vi "State_Machine.vi"(8 "error in (no error)":errorcluster caption="entrée d'erreur (pas d'erreur)", 11 "Get_Voltage en entrée":refnum<class "Get_SN_DB_AIS.lvclass">) -> (0 "error out":errorcluster caption="sortie d'erreur", 2 "Json_String":string, 3 "Get_Voltage en sortie":refnum<class "Get_SN_DB_AIS.lvclass">)   [LabVIEW 2020, in "Library Test.lvlib" / "Get_SN_DB_AIS.lvclass"]
uses:
  Get_SN_DB_AIS.lvclass
  C:/Users/ngarcin/OneDrive - Altyor/Standard TB/Suite TB45/Class/Test/Test (Default)/Test (Default).lvclass
  Database/Database Altyor/Database Altyor.lvclass
  C:/Users/ngarcin/OneDrive - Altyor/Standard TB/Suite TB45/Class/Database/Database drivers/Database Drivers.lvclass
  Commun VI/TypeDef/Variable Printable.ctl
  JSON API/JSON Value/Set from JSON string.vi
  Instrument/Instrument (Default)/Class Instrument (Default).lvclass
  JSON API/JSON Value/JSON Value.lvclass
  JSON API/Variant JSON/Variant JSON.lvlib
  JSON API/Get Polymorphic/JSON GetSet.lvlib
  Commun VI/Library Commun.lvlib
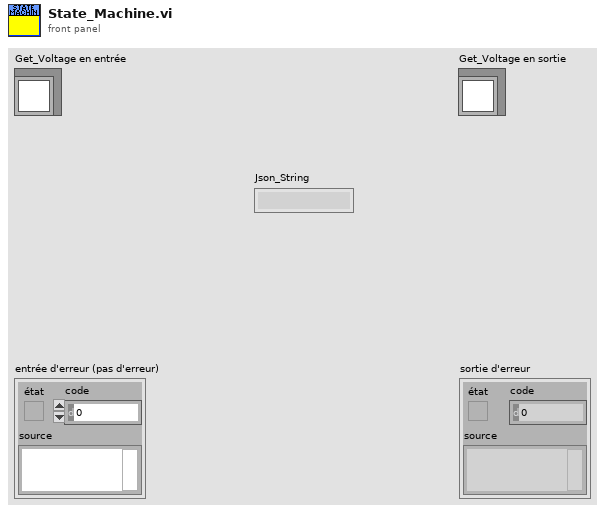
[diagram p1: front panel]
types:
  T1 = typedef "Variable Printable.ctl" = string
  T2 = enum16{"Get Variable", "Get All Variables", "Set Variable", "Delete Variable", "Delete All Variable"}
  T3 = cluster{"Connection Name ODBC":string, "DatabaseName":string, "Condition":string, "Type Data ":enum16{"Data Product", "Data Test"}, "Database Altyor":refnum<class "Database Altyor.lvclass">}
  T4 = cluster{"idTest":u32, "CreationDate":string, "EndOfProduction":string, "OrderNumber":string, "Batch":string, "ProductName":string, "PartNumber":string, "SerialNumber":string, "Operator":string, "Result":string, "AdditionalInformation":string}[]
  T5 = cluster{"idTest":u32, "CreationDate":string, "EndOfProduction":string, "OrderNumber":string, "Batch":string, "ProductName":string, "PartNumber":string, "SerialNumber":string, "Operator":string, "Result":string, "AdditionalInformation":string}
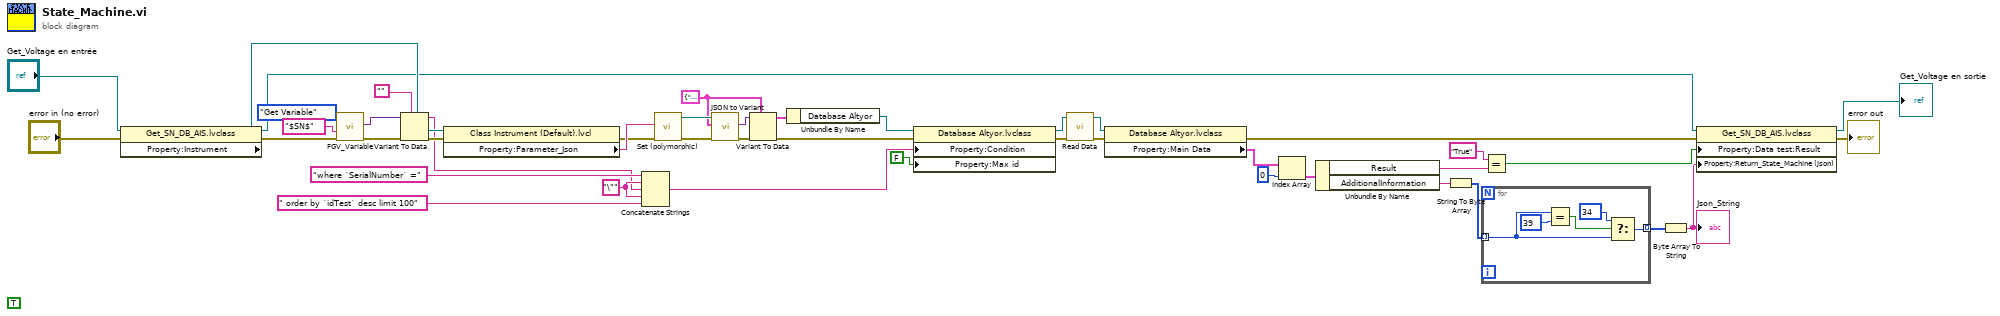
[diagram p0: block diagram]
diagram:
  w18 = "\"" ("chaîne")
  (unwired) TRUE ("Max id")
  w40 = T3 {"Connection Name ODBC"="", "DatabaseName"="", "Condition"="", "Type Data "=enum."Data Product", "Database Altyor"=refnum} ("Parameter")
  n1 = property class="Get_SN_DB_AIS.lvclass"(reference="Get_Voltage en entrée", error in="error in (no error)") -> (reference out=w9:refnum<class "Get_SN_DB_AIS.lvclass">, error out=w25:errorcluster, "Property:Instrument"=w23:refnum<class "Class Instrument (Default).lvclass">)
  n2 = call "FGV_Variable.vi"("error in (no error)"=w25, "Variable"=T1 "$SN$", "Function"=T2."Get Variable") -> ("error out"=w24:errorcluster, "Data Out"=w22:variant)  [unwired: 6 in, 1 out]
  n3 = Variant To Data(error in=w24, type="", Variant=w22) -> (data=w17:string, error out=w21:errorcluster)
  n4 = property class="Class Instrument (Default).lvcl"(reference=w23, error in=w21) -> (error out=w38:errorcluster, "Property:Parameter_Json"=w39:string)  [unwired: 1 out]
  n5 = Concatenate Strings("where `SerialNumber` =" ("chaîne"), w18, w17, w18, " order by `idTest` desc limit 100" ("chaîne")) -> (w16:string)
  n6 = call-poly "Set (polymorphic).vi"("error in (no error)"=w38, "JSON stream"=w39) -> ("error out"=w42:errorcluster, "JSON Value out"=w44:refnum<class "JSON Value.lvclass">)  [unwired: 7 in, 1 out]
  n7 = call "JSON to Variant.vi"("error in (no error)"=w42, "Variant (Data Type)"=w40, "JSON Value"=w44) -> ("error out"=w43:errorcluster, "Variant out"=w41:variant)  [unwired: 7 in]
  n8 = Variant To Data(error in=w43, type=w40, Variant=w41) -> (data=w37:T3, error out=w29:errorcluster)
  n9 = Unbundle By Name(w37) -> ("Database Altyor"=w28:refnum<class "Database Altyor.lvclass">)
  n10 = property class="Database Altyor.lvclass"(reference=w28, error in=w29, "Property:Condition"=w16, "Property:Max id"=FALSE ("Max id")) -> (reference out=w34:refnum<class "Database Altyor.lvclass">, error out=w33:errorcluster)
  n11 = call-dynamic "Read Data.vi"("error in (no error)"=w33, "Database Altyor en entrée"=w34) -> ("error out"=w31:errorcluster, "Database Altyor en sortie"=w32:refnum<class "Database Altyor.lvclass">)  [unwired: 8 in]
  n12 = property class="Database Altyor.lvclass"(reference=w32, error in=w31) -> (error out=w7:errorcluster, "Property:Main Data"=w14:T4)  [unwired: 1 out]
  n13 = Index Array(array=w14, index=0 ("indice")) -> (element=w12:T5)
  n14 = Unbundle By Name(w12) -> ("Result"=w11:string, "AdditionalInformation"=w2:string)
  n15 = String To Byte Array(string=w2) -> (unsigned byte array=w4:u8[])
  n16 = for {
    tunnel: w4 -> [w46] mode=indexing
    tunnel: [w45] -> w3 mode=indexing
    n17 = Equal?(x=w46, y=u8 39) -> (x = y?=w48:bool)
    n18 = Select(t=u8 34 ("y"), s=w48, f=w46) -> (s? t:f=w45:u8)
  }
  n19 = Equal?(x="True", y=w11) -> (x = y?=w8:bool)
  n20 = Byte Array To String(unsigned byte array=w3) -> (string=w1:string)
  "Json_String" <- w1
  n21 = property class="Get_SN_DB_AIS.lvclass"(reference=w9, error in=w7, "Property:Data test:Result"=w8, "Property:Return_State_Machine (Json)"=w1) -> (reference out=→"Get_Voltage en sortie":refnum<class "Get_SN_DB_AIS.lvclass">, error out=→"error out":errorcluster)
